vi "APP_User Event(FGV).vi"(6 "User Event Method(Put Event)":T2=enum."Put Event", 8 "error in":errorcluster, 10 "Subpanel Name":T1, 11 "User Event Data":T3) -> (0 "error out":errorcluster, 3 "User Event Ref.":refnum<user-event>)   [LabVIEW 2018, in "Application 1.lvlib"]
uses:
  Application 1.lvlib
  Data Def/App_User Event Data.ctl
  Data Def/App_User Event Method.ctl
  Data Def/App_Subpanel Name.ctl
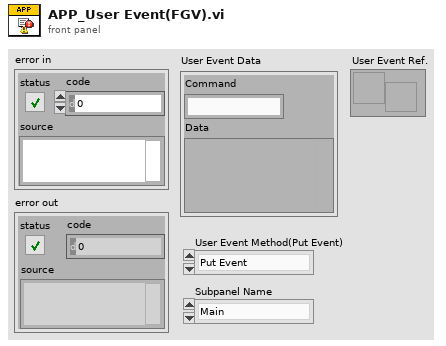
[diagram p1: front panel]
types:
  T1 = typedef "Application 1.lvlib/App_Subpanel Name.ctl" = enum16{"Main", "Menu", "User Registering", "User Setting", "Monitor", "Traning Mode", "Query Data", "Connect Setting"}
  T2 = typedef "Application 1.lvlib/App_User Event Method.ctl" = enum16{"Initialize", "Put Event", "Get Ref.", "Release"}
  T3 = typedef "Application 1.lvlib/App_User Event Data.ctl" = cluster{"Command":string, "Data":variant}
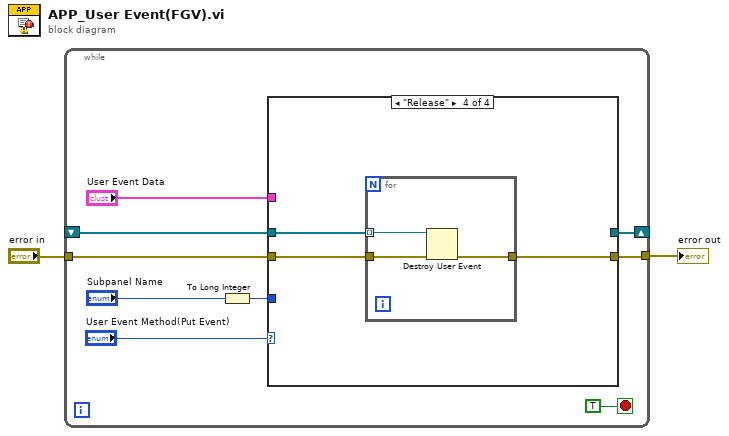
[diagram p0: block diagram]
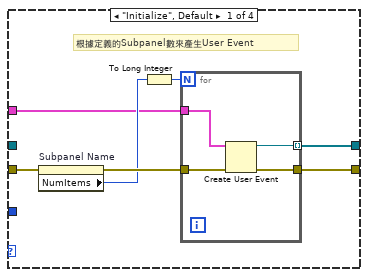
[diagram p2: hidden frame]
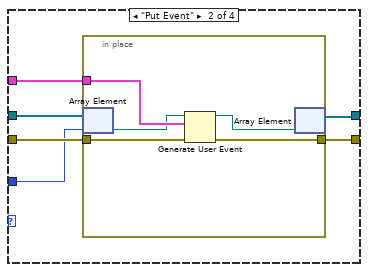
[diagram p3: hidden frame]
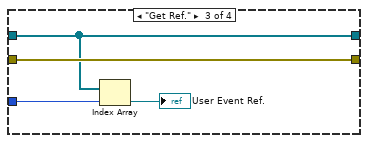
[diagram p4: hidden frame]
diagram:
  n1 = while {
    tunnel: "error in" -> [w9]
    shift-right: [w8] -> _
    shift-left: _ -> [w6]
    tunnel: [w5] -> w1
    stop <- TRUE stop-if-true
    n2 = To Long Integer(number="Subpanel Name") -> (32bit integer=w3:i32)
    n3 = case shown="\"Release\"" "User Event Method(Put Event)" {
      tunnel: w9 -> [w18 w27 w37 w40]
      tunnel: [w16 w25 w37 w38] -> w5
      tunnel: [w13 w24 w36 _] -> w8
      tunnel: "User Event Data" -> [w12 w26 _ _]
      tunnel: w6 -> [_ w28 w36 w39]
      tunnel: w3 -> [_ w23 w35 _]
      frame "Initialize", Default {
        # "根據定義的Subpanel數來產生User Event"
        n4 = property on="Subpanel Name" class="Enum (strict)"(error in=w18) -> (error out=w17:errorcluster, "NumItems"=w14:u32)  [unwired: 1 in, 1 out]
        n5 = To Long Integer(number=w14) -> (32bit integer=w15:i32)
        n6 = for {
          N: w15 -> [_]
          tunnel: w17 -> [w22]
          tunnel: w12 -> [w21]
          tunnel: [w20] -> w16
          tunnel: [w19] -> w13 mode=indexing
          n7 = Create User Event(user event datatype=w21, error in=w22) -> (user event=w19:refnum<user-event>, error out=w20:errorcluster)
        }
      }
      frame "Put Event" {
        n8 = in-place {
          in-place-border: w27 -> [w33]
          in-place-border: w26 -> [w32]
          in-place-border: [w30] -> w25
          n9 = in-place-array #1(w28, w23) -> (w31:refnum<user-event>)
          n10 = Generate User Event(user event=w31, event data cluster=w32, error in=w33) -> (user event out=w29:refnum<user-event>, error out=w30:errorcluster)  [unwired: 1 in]
          n11 = in-place-array #1(w29) -> (w24:refnum<user-event>[])  [unwired: 1 out]
        }
      }
      frame "Get Ref." {
        n12 = Index Array(array=w36, index=w35) -> (element=→"User Event Ref.":refnum<user-event>)
      }
      frame "Release" {
        n13 = for {
          tunnel: w40 -> [w42]
          tunnel: w39 -> [w43] mode=indexing
          tunnel: [w41] -> w38
          n14 = Destroy User Event(user event=w43, error in=w42) -> (error out=w41:errorcluster)
        }
      }
    }
  }
  "error out" <- w1
